vi "Create User Key.vi"(8 "error in (no error)":errorcluster, 11 "Server Fixture in":refnum<class "Server Fixture.lvclass">) -> (0 "error out":errorcluster, 3 "Server Fixture out":refnum<class "Server Fixture.lvclass">)   [LabVIEW 2013, in "libssh2_integration_tests.lvlib" / "Server Fixture.lvclass"]
uses:
  Server Fixture.lvclass
  Server Fixture.lvclass/Server Fixture.ctl
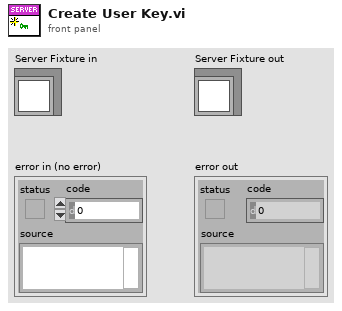
[diagram p1: front panel]
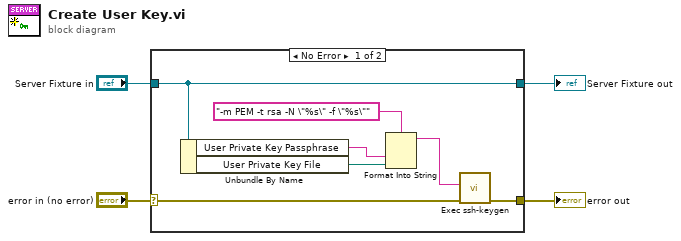
[diagram p0: block diagram]
diagram:
  n1 = case shown="No Error" "error in (no error)" {
    selector: "error in (no error)" -> [w6 w13]
    tunnel: [w5 w13] -> w3
    tunnel: [w7 w12] -> w1
    tunnel: "Server Fixture in" -> [w7 w12]
    frame No Error {
      n2 = Unbundle By Name(w7) -> ("User Private Key Passphrase"=w8:string, "User Private Key File"=w9:path)
      n3 = Format Into String(format string="-m PEM -t rsa -N \"%s\" -f \"%s\"" ("arguments"), w8, w9) -> (resulting string=w10:string)  [unwired: 2 in, 1 out]
      n4 = call "Exec ssh-keygen.vi"("error in (no error)"=w6, "arguments"=w10) -> ("error out"=w5:errorcluster)  [unwired: 9 in]
    }
    frame Error {
    }
  }
  "error out" <- w3
  "Server Fixture out" <- w1
